vi "DataFGV.vi"(8 "error in (no error)":errorcluster, 10 "AllData in":T1, 11 "Command":T4) -> (0 "error out":errorcluster, 2 "AllData out":T1)   [LabVIEW 2017]
uses:
  TypeDefs/DataFGVControl.ctl
  TypeDefs/allData.ctl
  TypeDefs/dataOut.ctl
  TypeDefs/dataIn.ctl
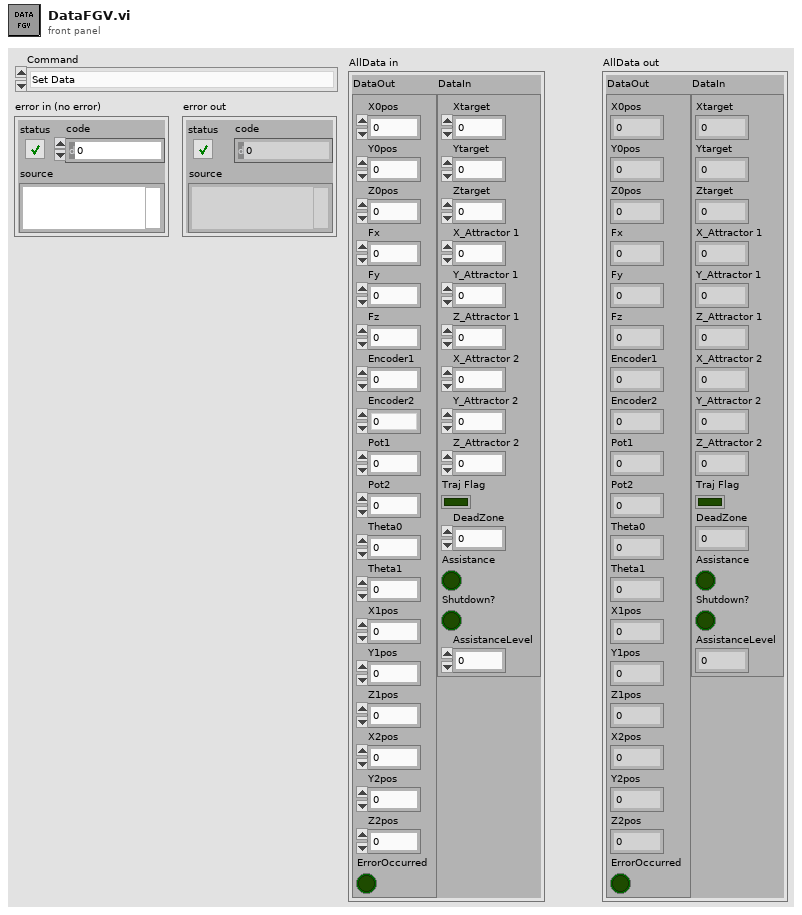
[diagram p1: front panel]
types:
  T1 = typedef "allData.ctl" = cluster{"DataOut":T2, "DataIn":T3}
  T2 = typedef "dataOut.ctl" = cluster{"X0pos":dbl, "Y0pos":dbl, "Z0pos":dbl, "Fx":dbl, "Fy":dbl, "Fz":dbl, "Encoder1":i32, "Encoder2":i32, "Pot1":dbl, "Pot2":dbl, "Theta0":dbl, "Theta1":dbl, "X1pos":dbl, "Y1pos":dbl, "Z1pos":dbl, "X2pos":dbl, "Y2pos":dbl, "Z2pos":dbl, "ErrorOccurred":bool}
  T3 = typedef "dataIn.ctl" = cluster{"Xtarget":dbl, "Ytarget":dbl, "Ztarget":dbl, "X_Attractor 1":dbl, "Y_Attractor 1":dbl, "Z_Attractor 1":dbl, "X_Attractor 2":dbl, "Y_Attractor 2":dbl, "Z_Attractor 2":dbl, "Traj Flag":bool, "DeadZone":dbl, "Assistance":bool, "Shutdown?":bool, "AssistanceLevel":dbl}
  T4 = typedef "DataFGVControl.ctl" = enum16{"Set Data", "Get Data"}
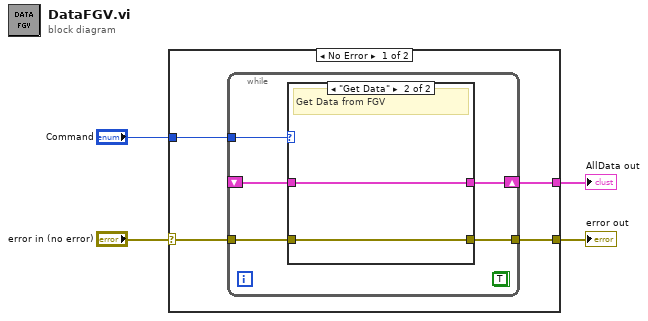
[diagram p0: block diagram]
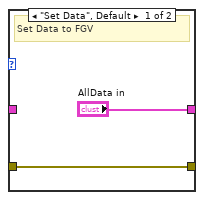
[diagram p2: hidden frame]
diagram:
  n1 = case shown="No Error" "error in (no error)" {
    selector: "error in (no error)" -> [w6 w19]
    tunnel: [w7 w19] -> w3
    tunnel: "Command" -> [w8 _]
    tunnel: [w5 _] -> w1
    frame No Error {
      n2 = while {
        tunnel: w8 -> [w13]
        tunnel: [w12] -> w7
        tunnel: w6 -> [w11]
        shift-right: [w10] -> w5
        shift-left: _ -> [w9]
        stop <- TRUE stop-if-true
        n3 = case shown="\"Get Data\"" w13 {
          tunnel: [w16 w18] -> w12
          tunnel: w11 -> [w16 w18]
          tunnel: ["AllData in" w17] -> w10
          tunnel: w9 -> [_ w17]
          frame "Set Data", Default {
            # "Set Data to FGV"
          }
          frame "Get Data" {
            # "Get Data from FGV"
          }
        }
      }
    }
    frame Error {
    }
  }
  "error out" <- w3
  "AllData out" <- w1
